vi "ShowHidden Strings Global.vi"() -> ()   [LabVIEW 2015]
panel:
  in  "Error Occurred":string="L'erreur %d est survenue lors de la tentative d'affichage des commandes et indicateurs masqués.  Vérifiez que le VI n'est ni réservé pour l'exécution ni verrouillé." caption="Une erreur est survenue"
  in  "None Found":string="Impossible de trouver des commandes ou indicateurs masqués." caption="Introuvable"
  in  "Undo Text":string="Afficher les commandes masquées" caption="Texte de Annuler"
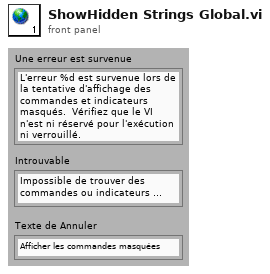
[diagram p1: front panel]
diagram:
